vi "Main Controller.vi"(8 "error in (no error)":errorcluster, 11 "Module_Refs":T1={"ModuleName"=enum."Controller", "Queue"=refnum, "user event"=refnum, "VI Refnum"=refnum, "ShowFP"=FALSE, "StatesTracking Enabled"=FALSE}) -> (0 "error out":errorcluster)   [LabVIEW 2019, in "Controller.lvlib"]
doc: "Main Module Template of the architecture. Use this as a template to integrate new independent processes into your application."
uses:
  Controller.lvlib
  Architecture/Typedefs/Enum_Module_Name.ctl
  Architecture/Architecture.lvlib
  Architecture/Typedefs/Message.ctl
  Architecture/Typedefs/Module References.ctl
  Typedefs/State Machine Data.ctl
  Architecture/Typedefs/Application Configuration.ctl
  Typedefs/Config.ctl
  Architecture/Modules/Module Template/SubVIs/Module Template Configuraton Extractor API.vi
  Architecture/Modules/Module Template/Typedefs/Config.ctl
  Architecture/Modules/Module Template/Module Template.lvlib
  <vilib>/event_ctls.llb/usereventprio.ctl
  Configuration Database/Typedefs/Messages.ctl
  Configuration Database/Configuration Database.lvlib
  Typedefs/State Machine States.ctl
panel:
  in  "Stop App":bool
  out "Message":string
  in  "Stop Module":bool
  # "#Architecture\n\nPlace inside this box all visible data."
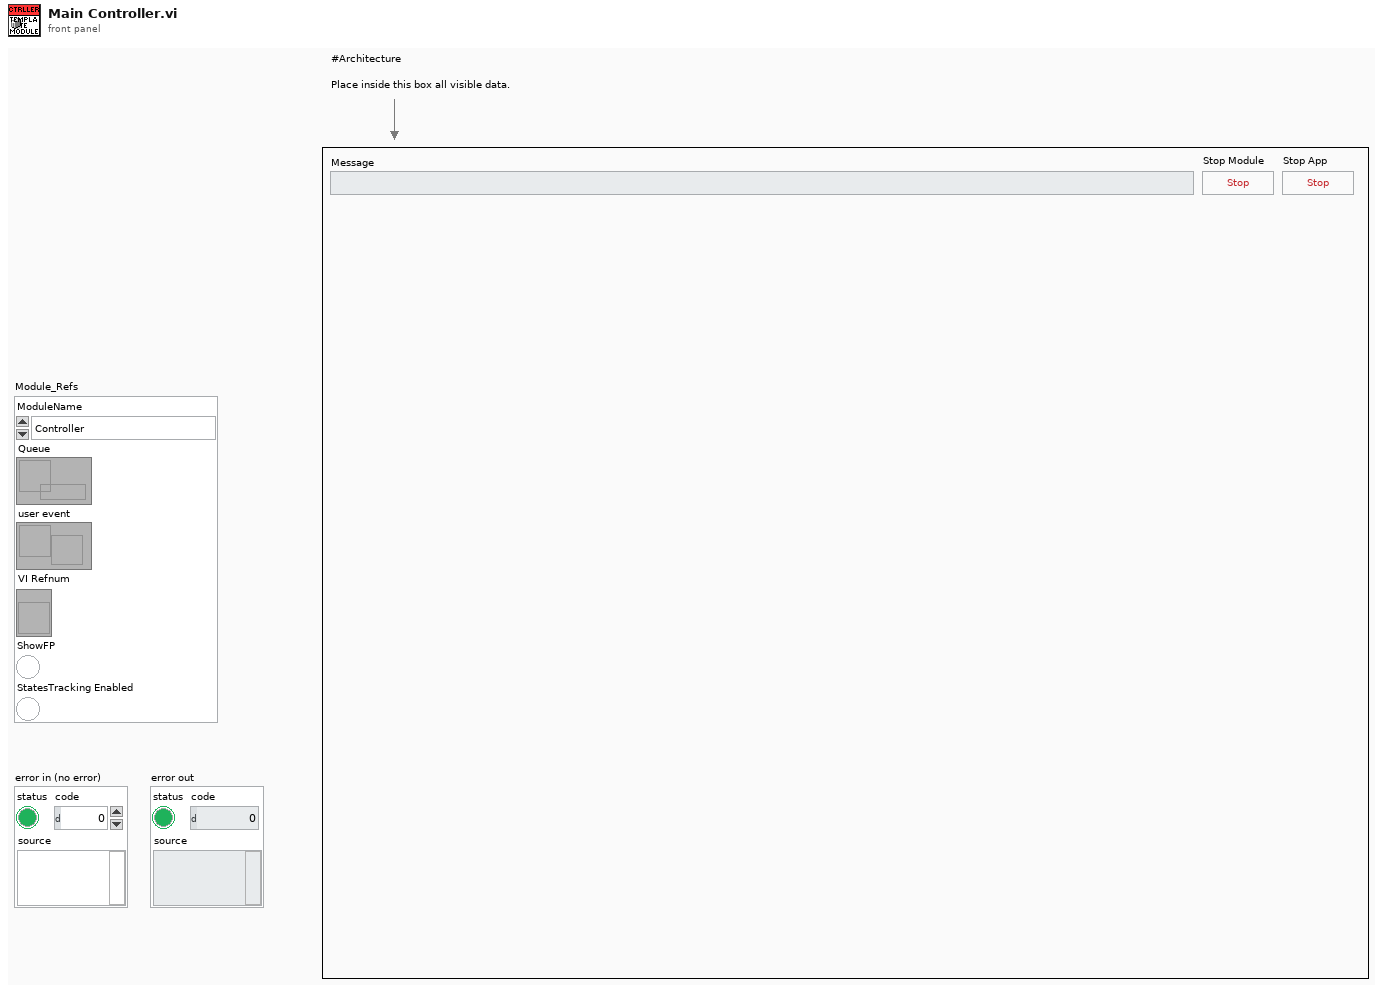
[diagram p1: front panel]
types:
  T1 = typedef "Architecture.lvlib/Module References.ctl" = cluster{"ModuleName":T2, "Queue":refnum<queue>, "user event":refnum<user-event>, "VI Refnum":refnum<vi>, "ShowFP":bool, "StatesTracking Enabled":bool}
  T2 = typedef "Architecture.lvlib/Enum_Module_Name.ctl" = enum16{"Configuration", "Error_Handler", "Log", "Database", "Controller", "User Console", "Display Console", "Sensor Interface"}
  T3 = typedef "Controller.lvlib/State Machine Data.ctl" = cluster{"Module_Refs":T1, "Response Data":variant, "Module Template Config":T4, "Curr State":T5, "Login Attempts":dbl}
  T4 = typedef "Controller.lvlib/Config.ctl" = cluster{"Module Enabled":bool}
  T5 = typedef "Controller.lvlib/State Machine States.ctl" = enum16{"Idle State", "Login State", "Balance Inquiry State", "Deposit State", "Withdrawal State", "Fast Cash State", "Terminate State", "Inactivity Timeout", "Wait For Transaction", "Add Balance"}
  T6 = enum32{"Invalid", "Standard", "Closed", "Hidden", "Minimized", "Maximized"}
  T7 = typedef "Configuration Database.lvlib/Messages.ctl" = enum16{"Welcome Message", "Login Message", "Idle Message", "Invalid Login Message", "Terminate Session Message", "Deposit Message", "Withdrawal Message", "Fast Cash $50 Message", "Withdrawal Complete Message", "Withdrawal Failed Message", "Balance Inquiry Message"}
  T8 = typedef "usereventprio.ctl" = enum32{"high priority", "normal priority"}
  T9 = typedef "Architecture.lvlib/Module Template.lvlib/Config.ctl" = cluster{"Module Enabled":bool}
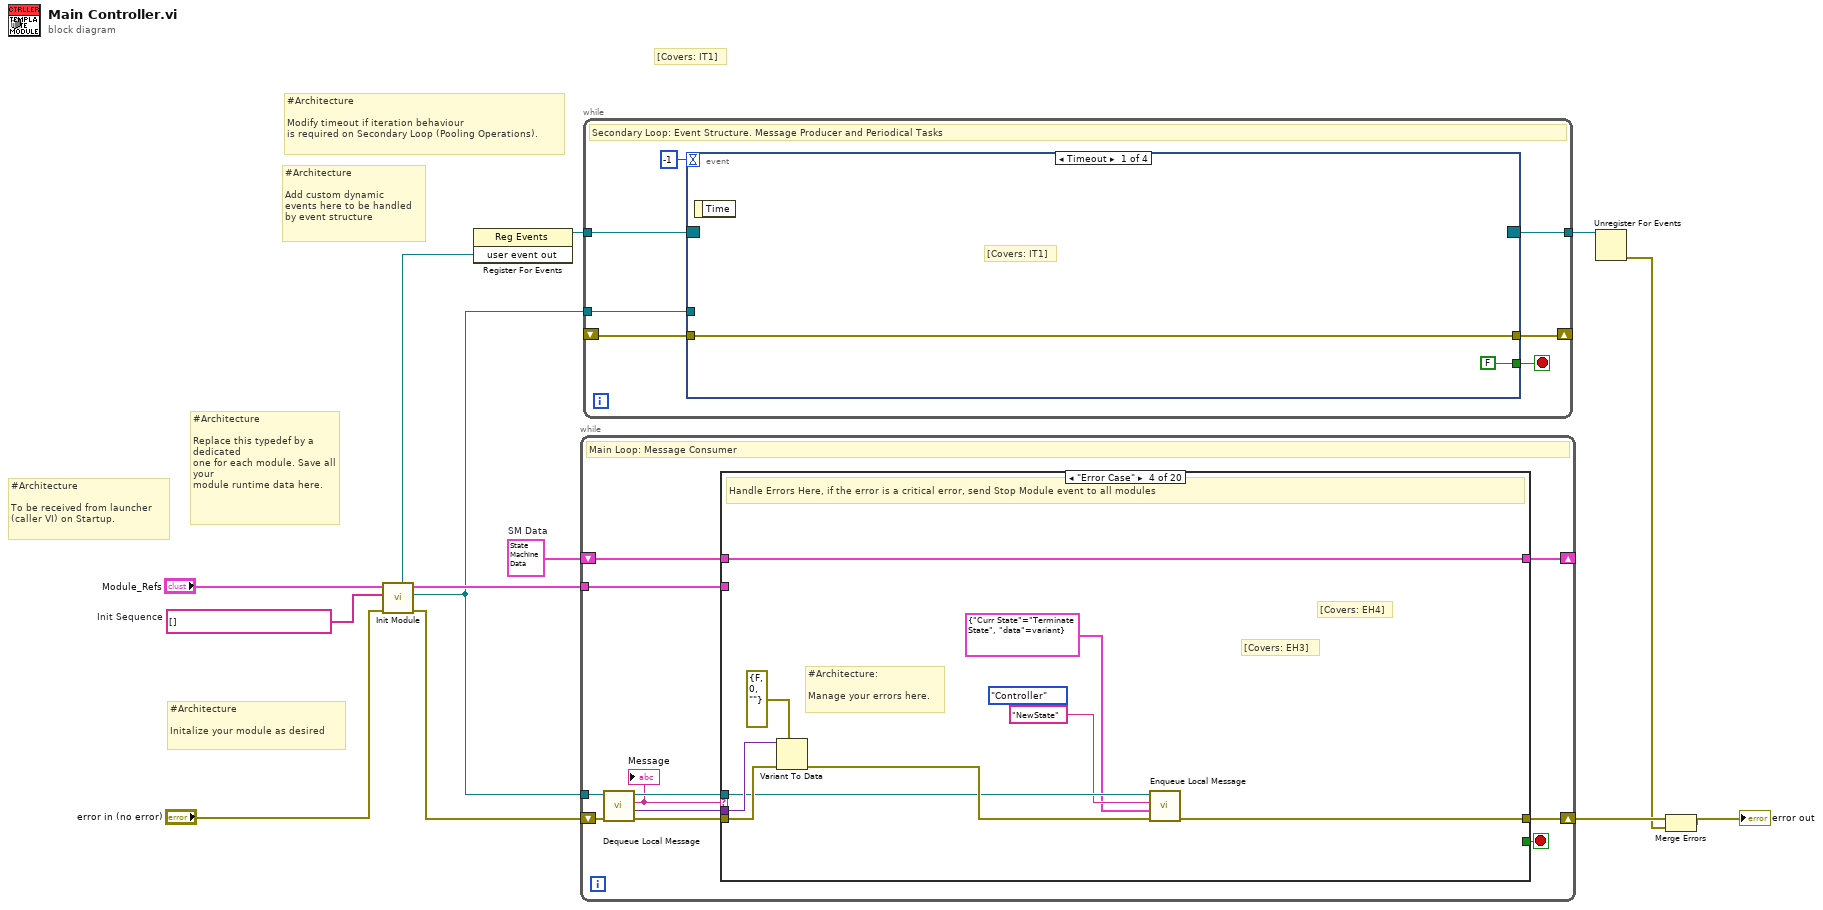
[diagram p0: block diagram]
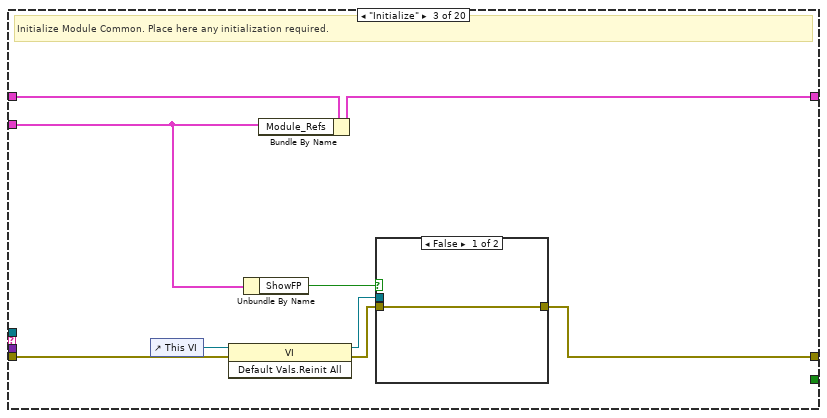
[diagram p4: hidden frame]
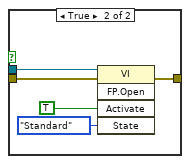
[diagram p5: hidden frame]
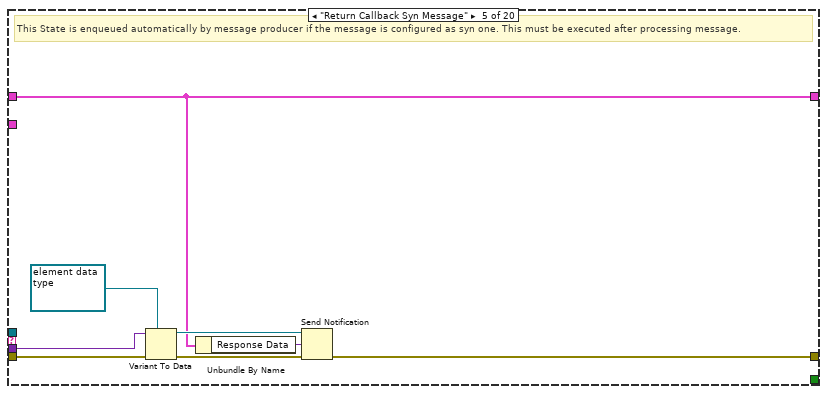
[diagram p6: hidden frame]
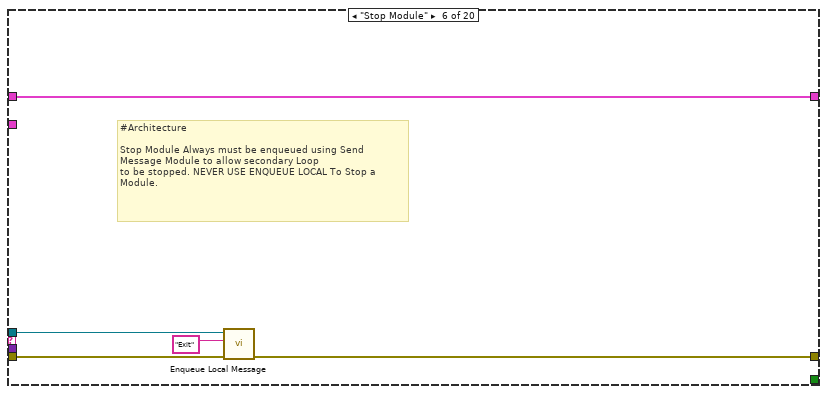
[diagram p7: hidden frame]
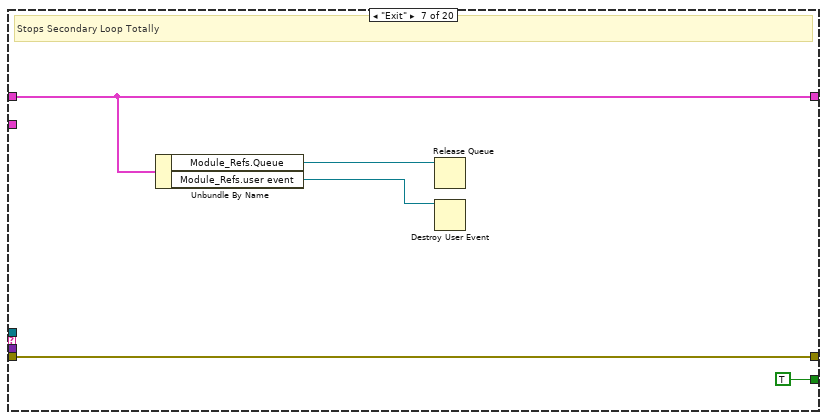
[diagram p8: hidden frame]
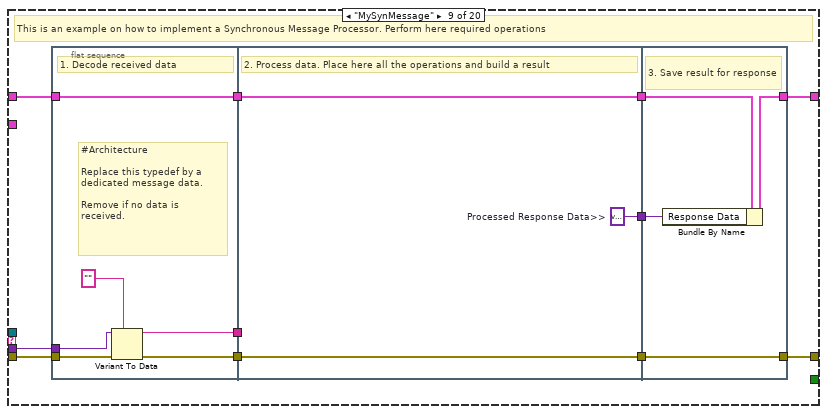
[diagram p10: hidden frame]
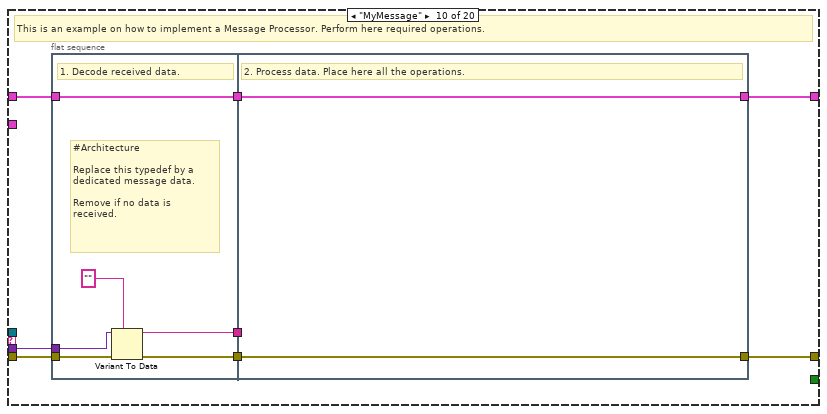
[diagram p11: hidden frame]
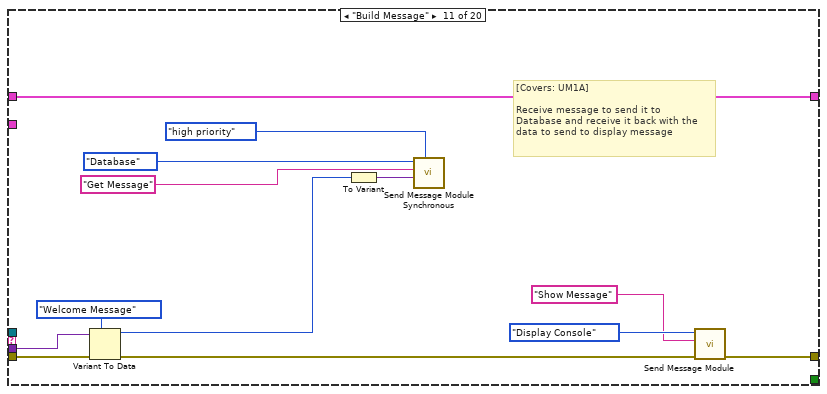
[diagram p12: hidden frame]
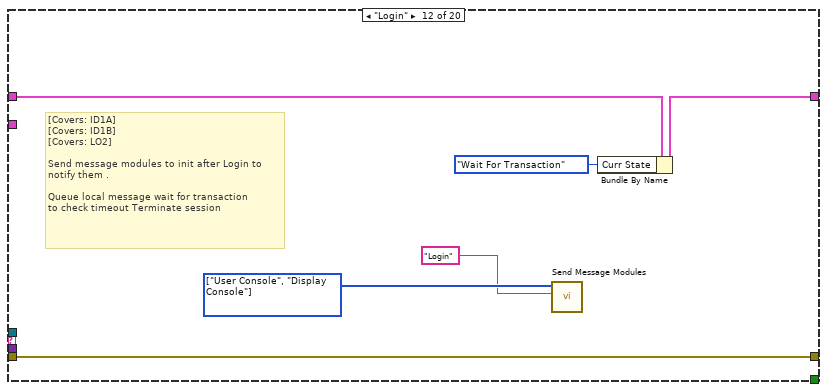
[diagram p13: hidden frame]
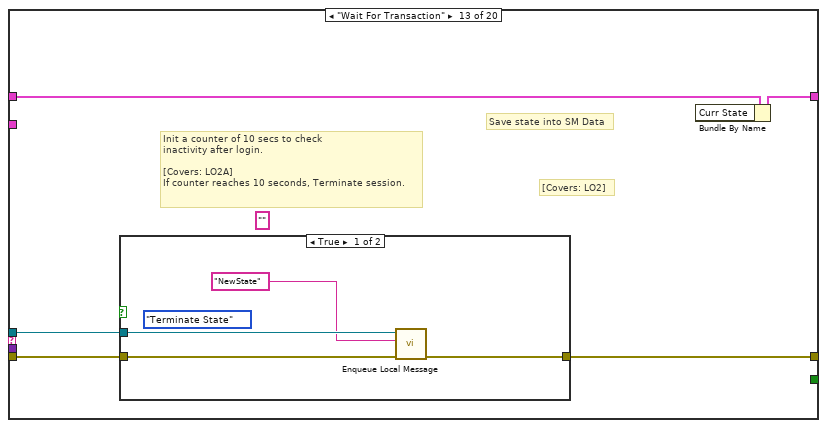
[diagram p14: hidden frame]
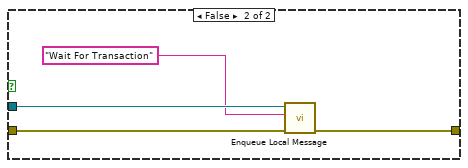
[diagram p15: hidden frame]
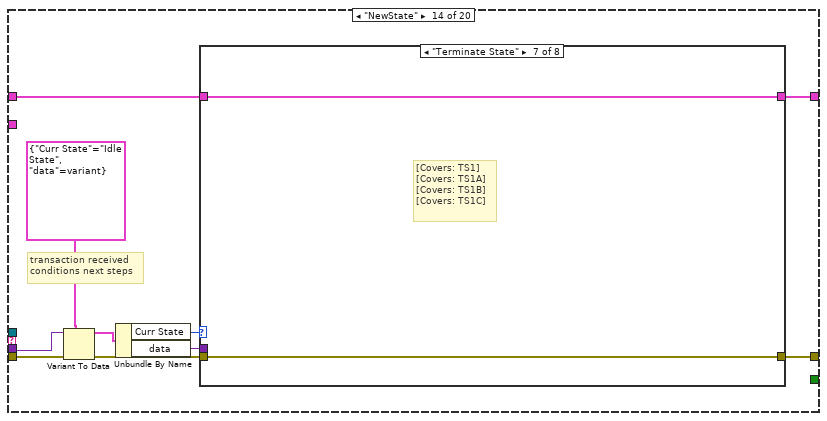
[diagram p16: hidden frame]
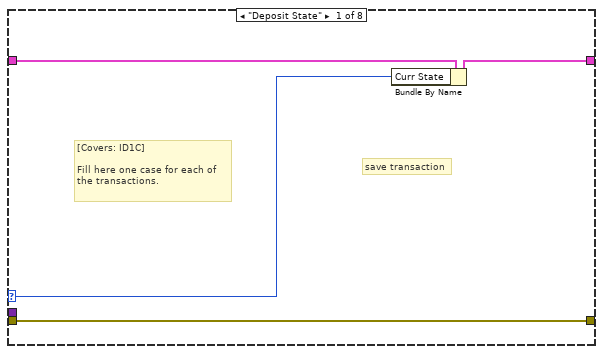
[diagram p17: hidden frame]
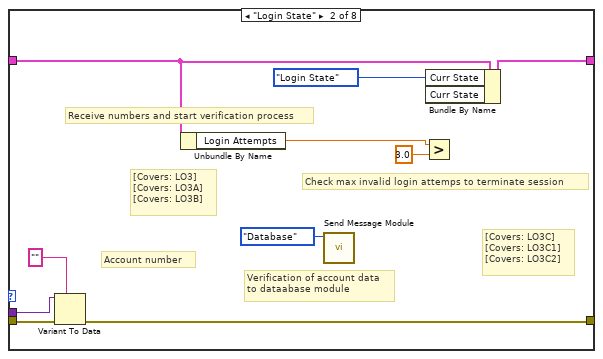
[diagram p18: hidden frame]
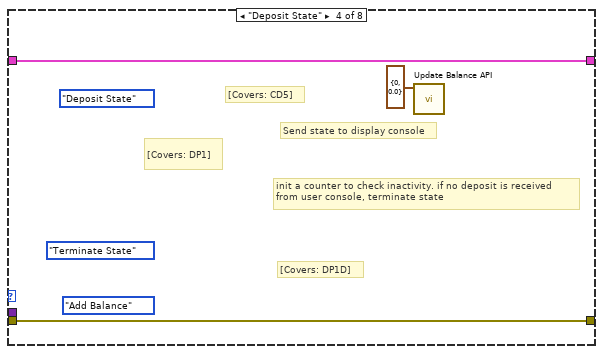
[diagram p20: hidden frame]
diagram:
  w10 = string[] []  # Init Sequence
  w13 = T3 {"Module_Refs"={"ModuleName"=enum."Controller", "Queue"=refnum, "user event"=refnum, "VI Refnum"=refnum, "ShowFP"=FALSE, "StatesTracking Enabled"=FALSE}, "Response Data"=variant, "Module Template Config"={"Module Enabled"=FALSE}, "Curr State"=enum."Idle State", "Login Attempts"=0.0}  # SM Data
  # "[Covers: IT1]"
  # "#Architecture\n\nModify timeout if iteration behaviour \nis required on Secondary Loop (Pooling Operations)."
  # "#Architecture\n\nAdd custom dynamic \nevents here to be handled \nby event structure"
  # "#Architecture\n\nInitalize your module as desired"
  # "#Architecture\n\nTo be received from launcher \n(caller VI) on Startup."
  # "#Architecture\n\nReplace this typedef by a dedicated \none for each module. Save all your \nmodule runtime data here."
  n1 = call "Init Module.vi"("error in (no error)"="error in (no error)", "Init Sequence"=w10, "Module Refs"="Module_Refs") -> ("error out"=w12:errorcluster, "queue out"=w1:refnum<queue>, "Module Refs Out"=w3:T1, "user event out"=w2:refnum<user-event>)  [unwired: 5 in]
  n2 = register-events(w2) -> (reference out=w9:refnum<event-registration>)  [unwired: 2 in, 1 out]
  n3 = while {
    shift-right: [w23] -> _
    shift-left: w13 -> [w24]
    shift-right: [w22] -> w7
    shift-left: w12 -> [w20]
    tunnel: w1 -> [w21]
    tunnel: w3 -> [w14]
    stop <- w15 stop-if-true
    # "Main Loop: Message Consumer"
    n4 = call "Dequeue Local Message.vi"("error in"=w20, "Msg queue in"=w21) -> ("error out"=w19:errorcluster, "Data"=w16:variant, "Message"=w17:string, "queue out"=w18:refnum<queue>)  [unwired: 6 in]
    "Message" <- w17
    n5 = case shown="\"Error Case\"" w17 {
      selector: w17 -> [_ _ _ _ _ _ _ _ _ _ _ _ _ _ _ w189 _ _ _ w221]
      tunnel: w24 -> [w26 w28 w37 w52 w54 w65 w68 w72 w83 w104 w125 w131 w136 w154 w188 w196 w201 w210 w212 w226]
      tunnel: [w26 w28 w35 w52 w54 w65 w68 w72 w82 w97 w125 w127 w132 w153 w188 w196 w201 w203 w212 w226] -> w23
      tunnel: w19 -> [w25 w27 w36 w51 w60 w64 w70 w71 w76 w100 w124 w130 w135 w152 w187 w193 w200 w209 w211 w225]
      tunnel: [w25 w27 w31 w47 w59 w63 w70 w71 w81 w103 w115 w130 w134 w145 w187 w190 w199 w204 w211 w215] -> w22
      tunnel: w18 -> [_ _ _ w46 _ w62 _ _ _ _ _ _ w133 _ _ w191 w198 _ _ w222]
      tunnel: w16 -> [_ _ _ w49 w57 _ _ _ w75 w99 w119 _ _ w150 _ w192 _ w208 _ w223]
      tunnel: [_ _ _ _ _ _ TRUE _ _ _ _ _ _ _ _ _ _ _ _ _] -> w15
      tunnel: w14 -> [_ _ w34 _ _ _ _ _ _ _ _ _ _ _ _ _ _ _ _ _]
      frame "--------State Machine Arquitechture Operations--------" {
      }
      frame "Idle", Default {
        # "Use this state to make iterations if required."
      }
      frame "Initialize" {
        # "Initialize Module Common. Place here any initialization required."
        n6 = control-ref of="This VI"() -> (w29:refnum<vi>)
        n7 = invoke class="VI" method="Default Vals.Reinit All"(reference=w29, error in=w36) -> (reference out=w32:refnum<vi>, error out=w33:errorcluster)  [unwired: 1 in, 1 out]
        n8 = Unbundle By Name(w34) -> ("ShowFP"=w30:bool)
        n9 = Bundle By Name(cluster=w37, "Module_Refs"=w34) -> (w35:T3)
        n10 = case shown="False" w30 {
          tunnel: w33 -> [w38 w43]
          tunnel: [w38 w42] -> w31
          tunnel: w32 -> [_ w41]
          frame False {
          }
          frame True {
            n11 = invoke class="VI" method="FP.Open"(reference=w41, error in=w43, "Activate"=TRUE ("Activate?"), "State"=T6."Standard") -> (error out=w42:errorcluster)  [unwired: 1 in, 4 out]
          }
        }
      }
      frame "Error Case" {
        (unwired) Enum_Module_Name."Controller" ("Target ModuleName In")
        # "[Covers: EH4]"
        # "[Covers: EH3]"
        # "#Architecture: \n\nManage your errors here."
        # "Handle Errors Here, if the error is a critical error, send Stop Module event to all modules"
        n12 = Variant To Data(error in=w51, type=errorcluster {"status"=FALSE, "code"=0, "source"=""} ("error constant"), Variant=w49) -> (error out=w50:errorcluster)  [unwired: 1 out]
        n13 = call "Enqueue Local Message.vi"("error in"=w50, "Data"=cluster{"Curr State":T5, "data":variant} {"Curr State"=enum."Terminate State", "data"=variant} ("data"), "Message"="NewState", "Msg queue in"=w46) -> ("error out"=w47:errorcluster)  [unwired: 6 in, 1 out]
      }
      frame "Return Callback Syn Message" {
        # "This State is enqueued automatically by message producer if the message is configured as syn one. This must be executed after processing message."
        n14 = Variant To Data(error in=w60, type=refnum<notifier> refnum ("notifier out"), Variant=w57) -> (data=w55:refnum<notifier>, error out=w58:errorcluster)
        n15 = Unbundle By Name(w54) -> ("Response Data"=w53:variant)
        n16 = Send Notification(notification=w53, notifier=w55, error in (no error)=w58) -> (error out=w59:errorcluster)  [unwired: 1 out]
      }
      frame "Stop Module" {
        # "#Architecture\n\nStop Module Always must be enqueued using Send Message Module to allow secondary Loop\nto be stopped. NEVER USE ENQUEUE LOCAL To Stop a Module."
        n17 = call "Enqueue Local Message.vi"("error in"=w64, "Message"="Exit", "Msg queue in"=w62) -> ("error out"=w63:errorcluster)  [unwired: 7 in, 1 out]
      }
      frame "Exit" {
        # "Stops Secondary Loop Totally"
        n18 = Unbundle By Name(w68) -> ("Module_Refs.Queue"=w67:refnum<queue>, "Module_Refs.user event"=w66:refnum<user-event>)
        n19 = Release Queue(queue=w67) -> ()  [unwired: 2 in, 3 out]
        n20 = Destroy User Event(user event=w66) -> ()  [unwired: 1 in, 1 out]
      }
      frame "--------------State Machine Custom States-------------" {
      }
      frame "MySynMessage" {
        # "This is an example on how to implement a Synchronous Message Processor. Perform here required operations"
        n21 = flat-sequence {
          tunnel: w76 -> [w87]
          tunnel: w83 -> [w89]
          tunnel: [w89] -> w80
          tunnel: [w85] -> w79
          tunnel: w75 -> [w86]
          tunnel: [w84] -> w74
          tunnel: w80 -> [w92]
          tunnel: w79 -> [w91]
          tunnel: [w92] -> w78
          tunnel: [w91] -> w77
          tunnel: w74 -> [_]
          tunnel: [w90] -> w73
          tunnel: [w95] -> w81
          tunnel: [w94] -> w82
          tunnel: w78 -> [w96]
          tunnel: w77 -> [w95]
          tunnel: w73 -> [w93]
          frame #0 {
            # "#Architecture\n\nReplace this typedef by a dedicated message data.\n\nRemove if no data is received."
            # "1. Decode received data"
            n22 = Variant To Data(error in=w87, type="", Variant=w86) -> (data=w84:string, error out=w85:errorcluster)
          }
          frame #1 {
            w90 = variant  # Processed Response Data>>
            # "2. Process data. Place here all the operations and build a result"
          }
          frame #2 {
            # "3. Save result for response"
            n23 = Bundle By Name(cluster=w96, "Response Data"=w93) -> (w94:T3)
          }
        }
      }
      frame "MyMessage" {
        # "This is an example on how to implement a Message Processor. Perform here required operations."
        n24 = flat-sequence {
          tunnel: w100 -> [w108]
          tunnel: w104 -> [w110]
          tunnel: [w110] -> w102
          tunnel: [w106] -> w101
          tunnel: w99 -> [w107]
          tunnel: [w105] -> w98
          tunnel: w102 -> [w111]
          tunnel: w101 -> [w112]
          tunnel: w98 -> [_]
          tunnel: [w112] -> w103
          tunnel: [w111] -> w97
          frame #0 {
            # "#Architecture\n\nReplace this typedef by a dedicated message data.\n\nRemove if no data is received."
            # "1. Decode received data."
            n25 = Variant To Data(error in=w108, type="", Variant=w107) -> (data=w105:string, error out=w106:errorcluster)
          }
          frame #1 {
            # "2. Process data. Place here all the operations."
          }
        }
      }
      frame "Build Message" {
        # "[Covers: UM1A]\n\nReceive message to send it to \nDatabase and receive it back with the \ndata to send to display message"
        n26 = Variant To Data(error in=w124, type=Messages."Welcome Message" ("Messages"), Variant=w119) -> (data=w117:T7, error out=w120:errorcluster)
        n27 = To Variant(anything=w117) -> (Variant=w116:variant)
        n28 = call "Send Message Module Synchronous.vi"("priority (normal)"=usereventprio."high priority", "Data"=w116, "Message"="Get Message", "Target ModuleName In"=Enum_Module_Name."Database") -> ()  [unwired: 6 in, 2 out]
        n29 = call "Send Message Module.vi"("Error In"=w120, "Message"="Show Message", "Target ModuleName In"=Enum_Module_Name."Display Console") -> ("error in (no error)"=w115:errorcluster)  [unwired: 8 in]
      }
      frame "Login" {
        w129 = T2[] [enum."User Console", enum."Display Console"] items=["Configuration", "Error_Handler", "Log", "Database", "Controller", "User Console", "Display Console", "Sensor Interface"] ("Target ModuleName In")
        # "[Covers: ID1A]   \n[Covers: ID1B]\n[Covers: LO2]\n\nSend message modules to init after Login to \nnotify them . \n\nQueue local message wait for transaction \nto check timeout Terminate session"
        n30 = call "Send Message Modules.vi"("Message"="Login", "Target ModuleName In"=w129) -> ()  [unwired: 9 in, 1 out]
        n31 = Bundle By Name(cluster=w131, "Curr State"=State_Machine_States."Wait For Transaction") -> (w127:T3)
      }
      frame "Wait For Transaction" {
        (unwired) "" ("Message")
        # "Save state into SM Data"
        # "[Covers: LO2]"
        # "Init a counter of 10 secs to check \ninactivity after login.\n\n[Covers: LO2A] \nIf counter reaches 10 seconds, Terminate session."
        n32 = case shown="True" {
          selector: _ -> [_ _]
          tunnel: w135 -> [w140 w144]
          tunnel: [w139 w143] -> w134
          tunnel: w133 -> [w138 w142]
          frame True {
            (unwired) State_Machine_States."Terminate State" ("Curr State")
            n33 = call "Enqueue Local Message.vi"("error in"=w140, "Message"="NewState", "Msg queue in"=w138) -> ("error out"=w139:errorcluster)  [unwired: 7 in, 1 out]
          }
          frame False {
            n34 = call "Enqueue Local Message.vi"("error in"=w144, "Message"="Wait For Transaction", "Msg queue in"=w142) -> ("error out"=w143:errorcluster)  [unwired: 7 in, 1 out]
          }
        }
        n35 = Bundle By Name(cluster=w136) -> (w132:T3)  [unwired: 1 in]
      }
      frame "NewState" {
        # "transaction received\nconditions next steps"
        n36 = Variant To Data(error in=w152, type=cluster{"Curr State":T5, "data":variant} {"Curr State"=enum."Idle State", "data"=variant}, Variant=w150) -> (data=w149:cluster{"Curr State":T5, "data":variant}, error out=w151:errorcluster)
        n37 = Unbundle By Name(w149) -> ("Curr State"=w147:T5, "data"=w146:variant)
        n38 = case shown="\"Terminate State\"" w147 {
          selector: w147 -> [w155 _ _ _ _ _ _ _]
          tunnel: w154 -> [w158 w163 w170 w173 w176 w179 w181 w186]
          tunnel: [w156 w162 w170 w173 w176 w179 w181 w186] -> w153
          tunnel: w151 -> [w157 w161 w169 w172 w175 w178 w180 w185]
          tunnel: w146 -> [_ w159 _ _ _ _ _ w182]
          tunnel: [w157 w160 w169 w172 w175 w178 w180 w184] -> w145
          frame "Deposit State" {
            # "[Covers: ID1C]\n\nFill here one case for each of \nthe transactions."
            # "save transaction"
            n39 = Bundle By Name(cluster=w158, "Curr State"=w155) -> (w156:T3)
          }
          frame "Login State" {
            # "Account number"
            # "[Covers: LO3C] \n[Covers: LO3C1] \n[Covers: LO3C2]"
            # "Check max invalid login attemps to terminate session"
            # "Verification of account data\nto dataabase module"
            # "[Covers: LO3] \n[Covers: LO3A] \n[Covers: LO3B]"
            # "Receive numbers and start verification process"
            n40 = Variant To Data(error in=w161, type="", Variant=w159) -> (error out=w160:errorcluster)  [unwired: 1 out]
            n41 = Unbundle By Name(w163) -> ("Login Attempts"=w168:dbl)
            n42 = call "Send Message Module.vi"("Target ModuleName In"=Enum_Module_Name."Database") -> ()  [unwired: 10 in, 1 out]
            n43 = Greater?(x=w168, y=3.0) -> ()  [unwired: 1 out]
            n44 = Bundle By Name(cluster=w163, "Curr State"=State_Machine_States."Login State") -> (w162:T3)  [unwired: 1 in]
          }
          frame "Balance Inquiry State" {
            # "[Covers: BI1] \n[Covers: BI1A] \n[Covers: BI1B]"
          }
          frame "Deposit State" {
            (unwired) State_Machine_States."Add Balance" ("Curr State")
            (unwired) State_Machine_States."Terminate State" ("Curr State")
            (unwired) State_Machine_States."Deposit State" ("Curr State")
            # "[Covers: CD5]"
            # "[Covers: DP1D]"
            # "init a counter to check inactivity. if no deposit is received \nfrom user console, terminate state"
            # "Send state to display console"
            # "[Covers: DP1]"
            n45 = call "Update Balance API.vi"("Update"=cluster{"Account Number":i32, "Udpate":dbl} {"Account Number"=0, "Udpate"=0.0}) -> ()  [unwired: 10 in, 1 out]
          }
          frame "Withdrawal State" {
            # "Send messages to all  modules to \ncover requirements"
            # "[Covers: WD1] \n[Covers: WD1A]  \n[Covers: WD1B] \n[Covers: WD1C] \n[Covers: WD1D]\n[Covers: WD1E]"
            n46 = call "Update Balance API.vi"("Update"=cluster{"Account Number":i32, "Udpate":dbl} {"Account Number"=0, "Udpate"=0.0}) -> ()  [unwired: 10 in, 1 out]
          }
          frame "Fast Cash State" {
            # "Send messages to all  modules to \ncover requirements"
            # "[Covers: FC1C] \n[Covers: FC1C1] \n[Covers: FC1C2]"
            # "[Covers: FC1] \n[Covers: FC1A] \n[Covers: FC1B] \n[Covers: FC1C] \n[Covers: FC1C1] \n[Covers: FC1C2]"
            n47 = call "Update Balance API.vi"("Update"=cluster{"Account Number":i32, "Udpate":dbl} {"Account Number"=0, "Udpate"=0.0}) -> ()  [unwired: 10 in, 1 out]
          }
          frame "Terminate State" {
            # "[Covers: TS1] \n[Covers: TS1A] \n[Covers: TS1B] \n[Covers: TS1C]"
          }
          frame "Add Balance" {
            # "Send balance to be added to user's account\n[Covers: DP1C3]"
            n48 = Variant To Data(error in=w185, type=0, Variant=w182) -> (error out=w184:errorcluster)  [unwired: 1 out]
          }
        }
      }
      frame "--------------Dynamic Events Messages----------------" {
      }
      frame "Message: Login", "Message: MyMessage", "Message: NewTransaction" {
        n49 = Match Pattern(string=w189, regular expression="Message: ") -> (after substring=w194:string)  [unwired: 1 in, 3 out]
        n50 = call "Enqueue Local Message.vi"("error in"=w193, "Data"=w192, "Message"=w194, "Msg queue in"=w191) -> ("error out"=w190:errorcluster)  [unwired: 6 in, 1 out]
      }
      frame "Message: Stop Module" {
        n51 = call "Enqueue Local Message.vi"("error in"=w200, "Message"="Stop Module", "Msg queue in"=w198) -> ("error out"=w199:errorcluster)  [unwired: 7 in, 1 out]
      }
      frame "Message: Load Config" {
        # "Get dedicated data for this module from \ngeneral DVR configuration and save it into \nSM Data to use it on runtime."
        # "Message used to receive configuration from a configuration module. Decode dedicated typedef and save it into SM Data"
        n52 = Variant To Data(error in=w209, type=refnum<data-value> refnum ("data value reference"), Variant=w208) -> (data=w206:refnum<data-value>, error out=w205:errorcluster)
        n53 = call-poly "Read Configuration API.vi"("error constant"=w205, "General Config DVR In"=w206) -> ("error out"=w204:errorcluster, "Module Template Config"=w202:T9)  [unwired: 8 in]
        n54 = Bundle By Name(cluster=w210, "Module Template Config"=w202) -> (w203:T3)
      }
      frame "------------Synchronous Event Messages--------------" {
      }
      frame "SynMessage: MySynMessage" {
        # "Use this case as a handler for Synchronous messages. This state queues a message for the desired"
        n55 = call "Extract Synchronous Data.vi"("error in 2"=w225, "Variant"=w223) -> ("error in"=w224:errorcluster, "Data Out"=w218:variant, "notifier out"=w213:refnum<notifier>)  [unwired: 7 in]
        n56 = Match Pattern(string=w221, regular expression="SynMessage: ") -> (after substring=w219:string)  [unwired: 1 in, 3 out]
        n57 = call "Enqueue Local Message.vi"("error in"=w224, "Data"=w218, "Message"=w219, "Msg queue in"=w222) -> ("error out"=w217:errorcluster, "queue out"=w216:refnum<queue>)  [unwired: 6 in]
        n58 = call "Enqueue Local Message.vi"("error in"=w217, "Data"=w213, "Message"="Return Callback Syn Message", "Msg queue in"=w216) -> ("error out"=w215:errorcluster)  [unwired: 6 in, 1 out]
      }
    }
  }
  n59 = while {
    tunnel: w9 -> [w233]
    tunnel: w1 -> [w230]
    tunnel: [w229] -> w8
    shift-right: [w227] -> _
    shift-left: _ -> [w228]
    stop <- w231 stop-if-true
    # "Secondary Loop: Event Structure. Message Producer and Periodical Tasks"
    n60 = event shown="[0] Timeout" {
      selector: w233 -> [_ _ _ _]
      dyn-events: [_ _ _ _] -> w229
      timeout: -1 -> [_ _ _ _]
      tunnel: [FALSE w242 TRUE _] -> w231
      tunnel: w230 -> [_ w247 w249 _]
      tunnel: w228 -> [w234 w246 w252 w254]
      tunnel: [w234 w245 w250 w253] -> w227
      event Timeout {
        # "[Covers: IT1]"
        n61 = event-data() -> ()  [unwired: 1 in, 1 out]
      }
      event User Event {
        # "Send message to local queue. \n(Message Consumer)"
        # "Processes an external event and enqueues a message to the local queue. It can be synchronous (with response) or NOT."
        n62 = event-data() -> ("syn"=w239:bool, "Message"=w241:string, "Data"=w244:variant)  [unwired: 1 in]
        n63 = Select(t="SynMessage: " ("string"), s=w239, f="Message: " ("string")) -> (s? t:f=w236:string)
        n64 = Concatenate Strings(w236, w241) -> (w243:string)
        n65 = call "Enqueue Local Message.vi"("error in"=w246, "Data"=w244, "Message"=w243, "Msg queue in"=w247) -> ("error out"=w245:errorcluster)  [unwired: 6 in, 1 out]
        n66 = Equal?(x=w241, y="Stop Module") -> (x = y?=w242:bool)
      }
      event "Stop Module": Value Change {
        n67 = event-data() -> ()  [unwired: 1 in, 1 out]
        n68 = call "Enqueue Local Message.vi"("error in"=w252, "Message"="Stop Module", "Msg queue in"=w249) -> ("error out"=w250:errorcluster)  [unwired: 7 in, 1 out]
      }
      event "Stop App": Value Change {
        w256 = TRUE  # All Modules
        # "Send Stop To All Modules"
        n69 = event-data() -> ()  [unwired: 1 in, 1 out]
        n70 = call "Send Message Modules.vi"("All Modules"=w256, "Error In"=w254, "Message"="Stop Module") -> ("error in (no error)"=w253:errorcluster)  [unwired: 8 in]
      }
    }
  }
  n71 = Unregister For Events(event registration refnum=w8) -> (error out=w6:errorcluster)  [unwired: 1 in]
  n72 = Merge Errors(w7, w6) -> (→"error out":errorcluster)
